vi "FilterOnNameInTree.vi"(8 "error in (no error)":errorcluster, 10 "Event Registration Refnum":refnum<event-registration>, 11 "TreeReference":refnum<vi>) -> (0 "error out":errorcluster)   [LabVIEW 2013, in "FindName Task_Manager.lvlib"]
doc: "Provides a mechanism to allow the user to specify a string to be searched for. Tree items containing a match continue to be displayed, while all non-matching items are removed from the tree. Also, a count of matching tree items is displayed, along with a count of all tree items."
uses:
  FindName Task_Manager.lvlib
  <vilib>/Utility/miscctls.llb/LVSelectionTypeDef.ctl
  <vilib>/Utility/error.llb/DialogType.ctl
panel:
  out "Found/Total =":string
  in  "Close":bool
  in  "NameToFilter":string caption="Filter ="
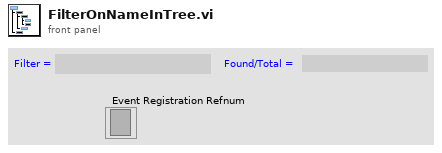
[diagram p1: front panel]
types:
  T1 = typedef "LVSelectionTypeDef.ctl" = cluster{"Selection Start":u32, "Selection End":u32}
  T2 = cluster{"Left Cell String":string, "Child Text":string[], "Child Tag":string, "Item Indent":i32, "Child Only?":bool, "Glyph Index":i32}[]
  T3 = typedef "DialogType.ctl" = u16
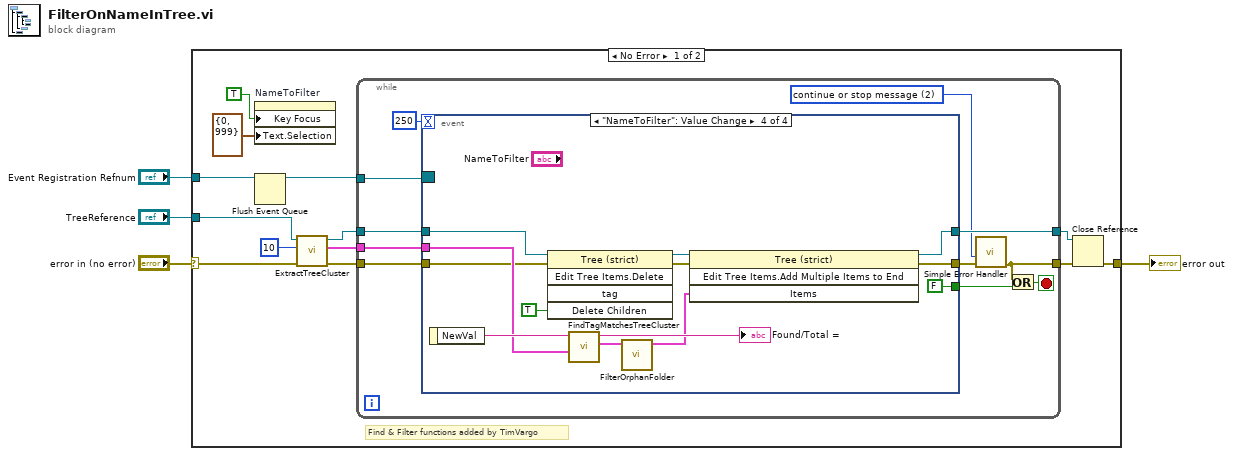
[diagram p0: block diagram]
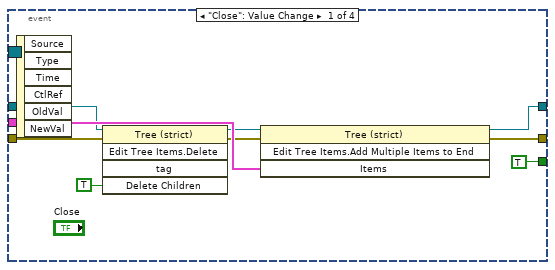
[diagram p2: hidden frame]
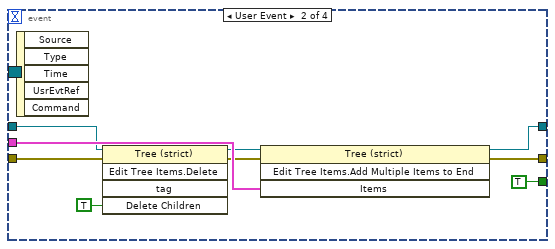
[diagram p3: hidden frame]
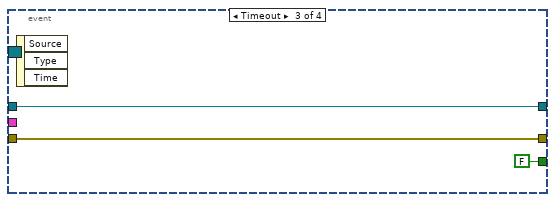
[diagram p4: hidden frame]
diagram:
  n1 = case shown="No Error" "error in (no error)" {
    selector: "error in (no error)" -> [w6 w63]
    tunnel: "TreeReference" -> [w10 _]
    tunnel: [w8 w63] -> w3
    tunnel: "Event Registration Refnum" -> [w7 _]
    frame No Error {
      # "Find & Filter functions added by TimVargo"
      n2 = property on="NameToFilter" class="Str"("Key Focus"=TRUE, "Text.Selection"=T1 {"Selection Start"=0, "Selection End"=999}) -> ()  [unwired: 2 in, 2 out]
      n3 = Flush Event Queue(0:w7) -> (8:w5:refnum<event-registration>)  [unwired: 5 in, 2 out]
      n4 = call "ExtractTreeCluster.vi"("error in (no error)"=w6, "NumberOfColumns"=10, "TreeReference"=w10) -> ("error out"=w11:errorcluster, "TreeCluster"=w13:T2, "TreeReference"=w12:refnum<vi>)  [unwired: 5 in, 1 out]
      n5 = while {
        tunnel: [w26] -> w17
        tunnel: w11 -> [w24]
        tunnel: w13 -> [w28]
        tunnel: [w20] -> w9
        tunnel: w12 -> [w27]
        tunnel: w5 -> [w23]
        stop <- w19 stop-if-true
        w18 = T3 2 items=["no dialog", "OK message", "continue or stop message", "OK message + warnings", "continue/stop + warnings"] ("type of dialog (OK msg:1)")
        n6 = event shown="[3] \"NameToFilter\": Value Change" {
          selector: w23 -> [_ _ _ _]
          dyn-events: _ -> [_ _ _ _]
          timeout: 250 -> [_ _ _ _]
          tunnel: w24 -> [w31 w40 w49 w54]
          tunnel: [w30 w39 w49 w53] -> w22
          tunnel: w28 -> [w37 w46 _ w57]
          tunnel: w27 -> [w34 w43 w48 w62]
          tunnel: [w33 w42 w48 w59] -> w26
          tunnel: [TRUE TRUE FALSE FALSE] -> w21
          event "Close": Value Change {
            n7 = event-data() -> ()  [unwired: 1 in, 6 out]
            n8 = invoke class="Tree (strict)" method="Edit Tree Items.Delete"(reference=w34, error in=w31, "Delete Children"=TRUE ("Delete Children?")) -> (reference out=w36:refnum<vi>, error out=w32:errorcluster)  [unwired: 2 in, 3 out]
            n9 = invoke class="Tree (strict)" method="Edit Tree Items.Add Multiple Items to End"(reference=w36, error in=w32, "Items"=w37) -> (reference out=w33:refnum<vi>, error out=w30:errorcluster)  [unwired: 1 in, 2 out]
          }
          event User Event {
            n10 = event-data() -> ()  [unwired: 1 in, 5 out]
            n11 = invoke class="Tree (strict)" method="Edit Tree Items.Delete"(reference=w43, error in=w40, "Delete Children"=TRUE ("Delete Children?")) -> (reference out=w45:refnum<vi>, error out=w41:errorcluster)  [unwired: 2 in, 3 out]
            n12 = invoke class="Tree (strict)" method="Edit Tree Items.Add Multiple Items to End"(reference=w45, error in=w41, "Items"=w46) -> (reference out=w42:refnum<vi>, error out=w39:errorcluster)  [unwired: 1 in, 2 out]
          }
          event Timeout {
            n13 = event-data() -> ()  [unwired: 1 in, 3 out]
          }
          event "NameToFilter": Value Change {
            n14 = event-data() -> ("NewVal"=w58:string)  [unwired: 1 in]
            n15 = invoke class="Tree (strict)" method="Edit Tree Items.Delete"(reference=w62, error in=w54, "Delete Children"=TRUE ("Delete Children?")) -> (reference out=w60:refnum<vi>, error out=w55:errorcluster)  [unwired: 2 in, 3 out]
            n16 = call "FindTagMatchesTreeCluster.vi"("TreeCluster"=w57, "NameToFind"=w58) -> ("TreeCluster"=w51:T2, "ResultString"=→"Found/Total =":string)  [unwired: 8 in]
            n17 = call "FilterOrphanFolder.vi"("TreeCluster"=w51) -> ("TreeCluster 2"=w50:T2)  [unwired: 10 in]
            n18 = invoke class="Tree (strict)" method="Edit Tree Items.Add Multiple Items to End"(reference=w60, error in=w55, "Items"=w50) -> (reference out=w59:refnum<vi>, error out=w53:errorcluster)  [unwired: 1 in, 2 out]
          }
        }
        n19 = call <vilib>:"Simple Error Handler.vi"("type of dialog (OK msg:1)"=w18, "error in (no error)"=w22) -> ("error out"=w20:errorcluster)  [unwired: 3 in, 4 out]
        n20 = Or(x=w20, y=w21) -> (x .or. y?=w19:bool)
      }
      n21 = Close Reference(reference=w17, error in (no error)=w9) -> (error out=w8:errorcluster)
    }
    frame Error {
    }
  }
  "error out" <- w3
